vi "OOP_test_main.vi"() -> ()   [LabVIEW 2013]
doc: "Main test automation program using object-oriented programming approach and a producer-consumer architecture."
uses:
  Classes/BaseProducer/IO Task Cluster.ctl
  Classes/BaseProducer/BaseProducer.lvclass
  Classes/BaseProducer/BaseProducer.lvclass/BaseProducer.ctl
panel:
  in  "Stop Button":bool
  in  "Abort":bool
  in  "Front Panel":T1(tab)
  in  "connection information":string="mySQL measurement data"
  in  "Initialize":bool
  in  "test state file path":path=path "C:/Users/Nathan/Documents/LV_testRig-Git/Data/state_sequence_10.txt"
  in  "table":string="10_op_point_test"
  in  "columns":string[](array[string])=["atmosphericP", "opPointDes", "opPointAct", "flameStatus", "dateTimeStamp", "staticP", "temperature", "dynamicP"]
  in  "IO Task Cluster":T2={"Dynamic P Tasks"="DynP_all_S6AI0-4", "AI Tasks"="AiTasks_TC_P_S3", "DIO Tasks"="MFCOutputEnable_S2P0L67", "AO Tasks"="MFCVoltageOut_S2AO0-3"}
  in  "Username":string="Nathan"
  in  "Password":string="admin"
  out "P ATM (psi abs)":dbl=14.424752317565863
  in  "Set P ATM":bool
  in  "Run":bool caption="Run Experiment"
  in  "Measure time (sec)":dbl=1.0
  in  "Back to Default":bool
  out "Remaining":dbl=1181.1679229736328 caption="Time Remaining (sec)"
  in  "End Cooldown":bool
  out "Relight Point":dbl[](array[numeric])=[0.7, 0.0, 2.0, 0.0]
  out "Des. Op. Pt.":dbl[](array[numeric]) caption="Des. Operating Point"
  out "Flame?":bool=TRUE
  out "Temperature Array (C)":dbl[](array[numeric])=[237.25402836473043, 230.0152646954811, 224.8556597910292, 144.771153562919, 153.15861192981532]
  out "Last Line Read":i16=11
  # "Flow Temp"
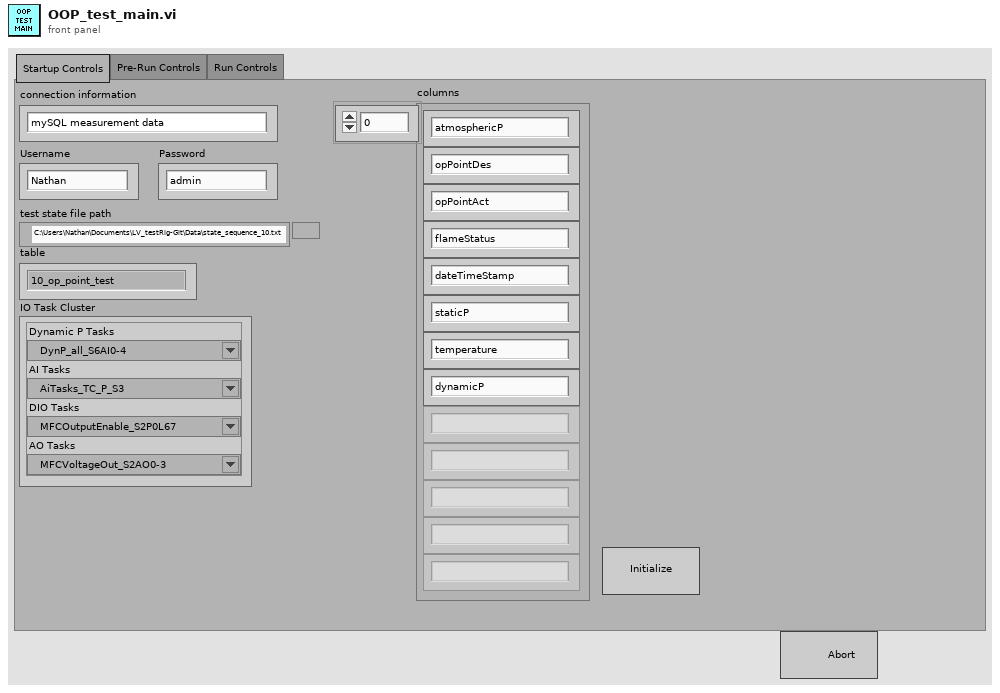
[diagram p1: front panel]
types:
  T1 = enum32{"Startup Controls", "Pre-Run Controls", "Run Controls"}
  T2 = typedef "BaseProducer.lvclass/IO Task Cluster.ctl" = cluster{"Dynamic P Tasks":refnum<k21>, "AI Tasks":refnum<k21>, "DIO Tasks":refnum<k21>, "AO Tasks":refnum<k21>}
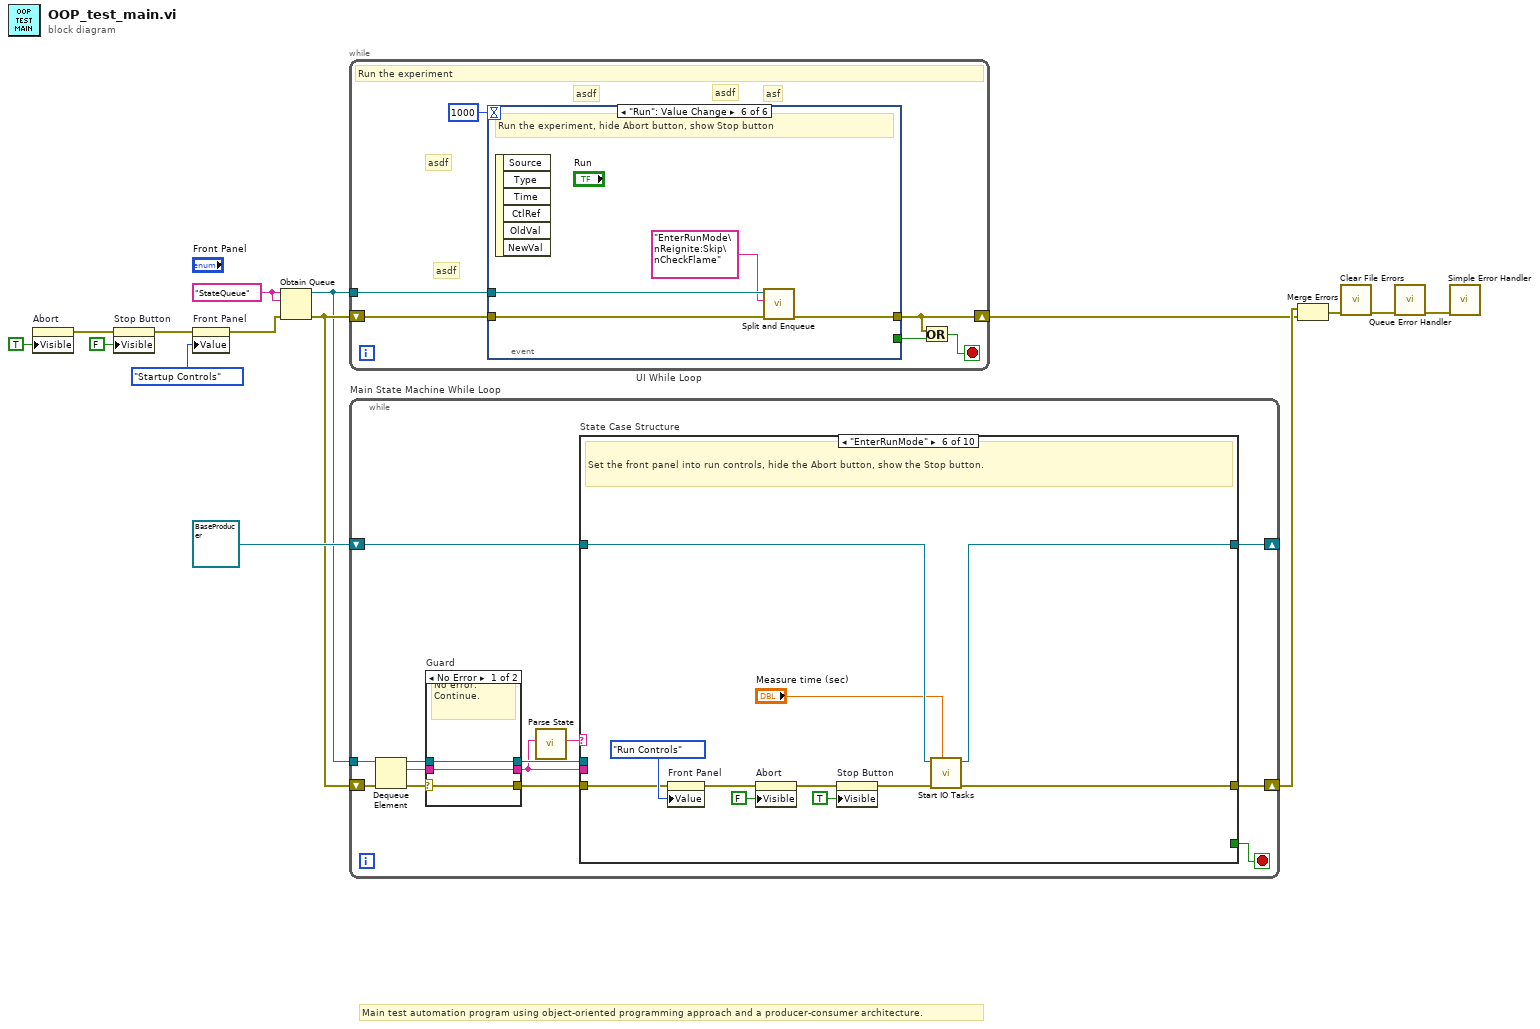
[diagram p0: block diagram]
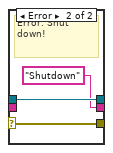
[diagram p2: hidden frame]
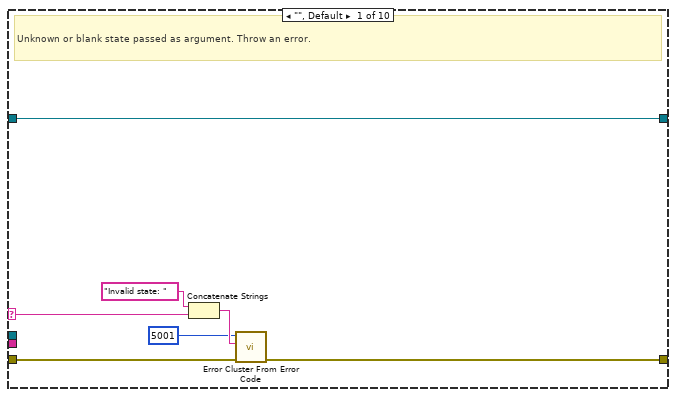
[diagram p3: hidden frame]
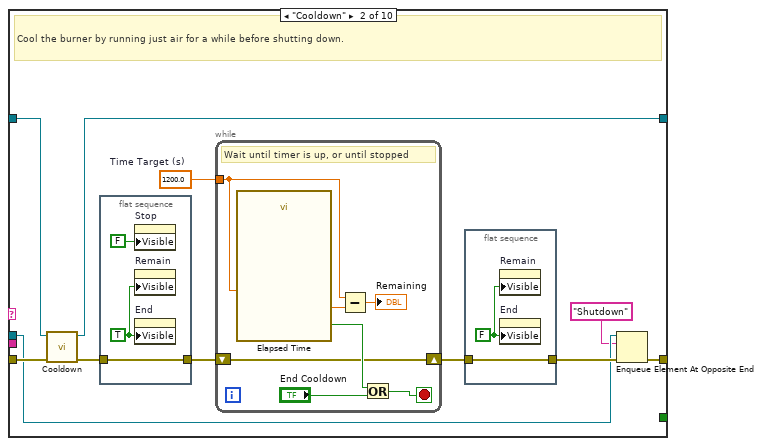
[diagram p4: hidden frame]
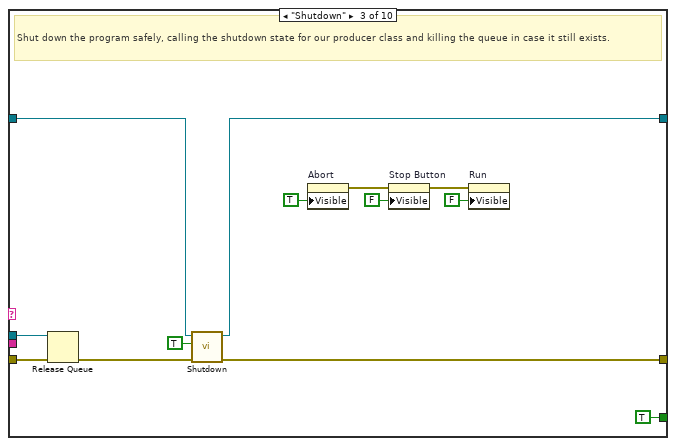
[diagram p5: hidden frame]
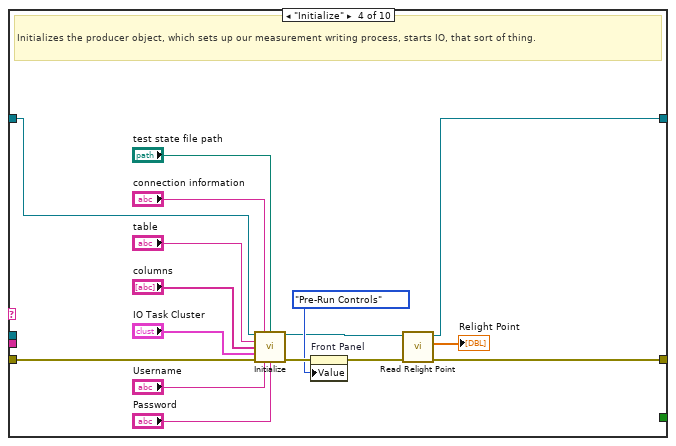
[diagram p6: hidden frame]
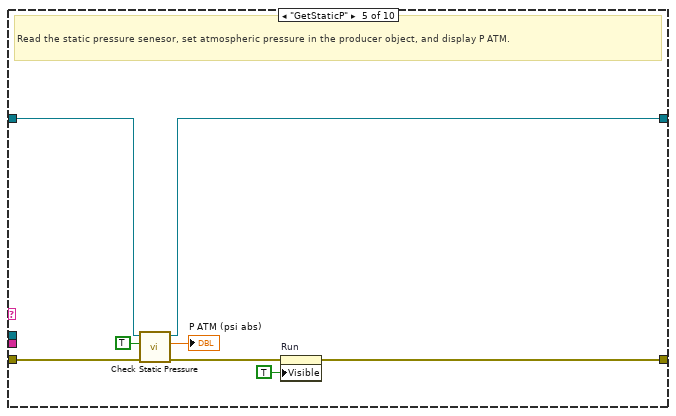
[diagram p7: hidden frame]
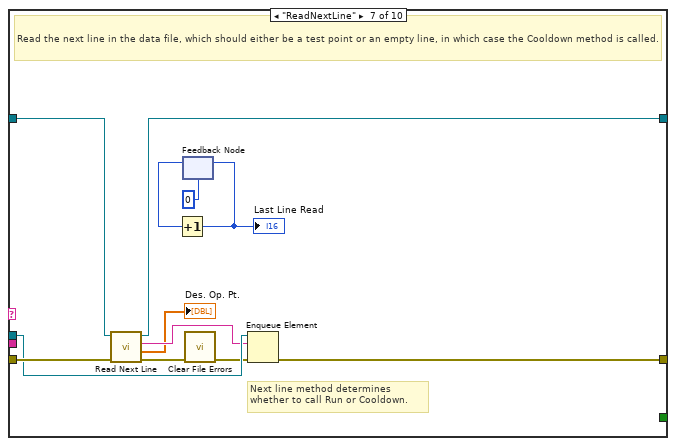
[diagram p8: hidden frame]
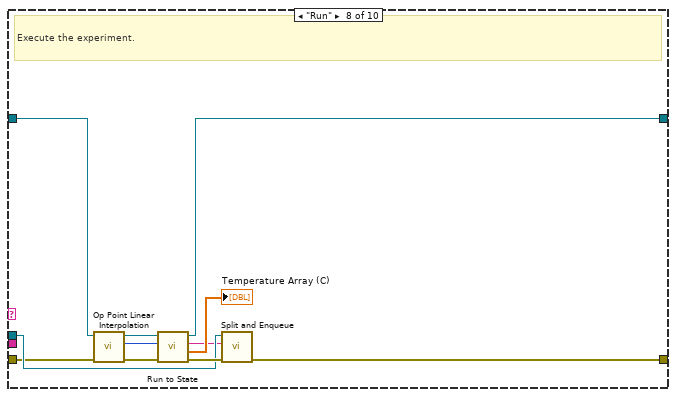
[diagram p9: hidden frame]
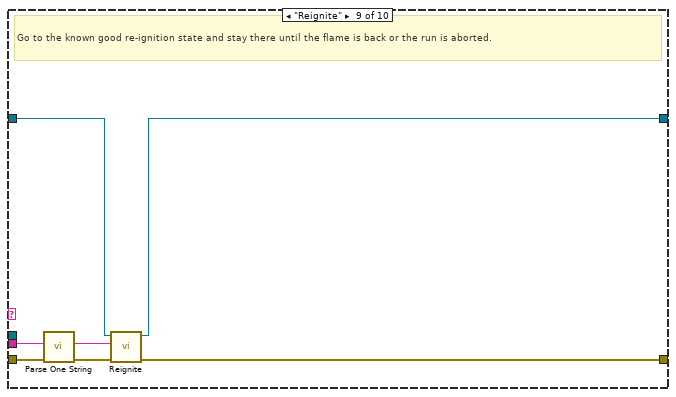
[diagram p10: hidden frame]
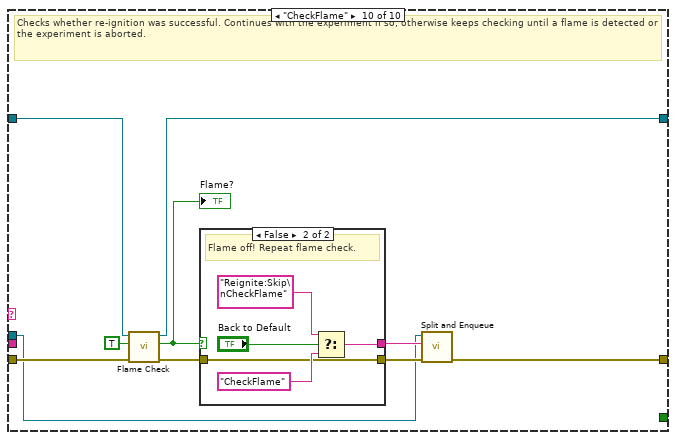
[diagram p11: hidden frame]
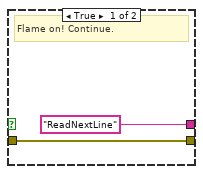
[diagram p12: hidden frame]
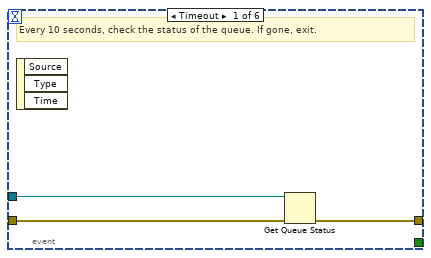
[diagram p13: hidden frame]
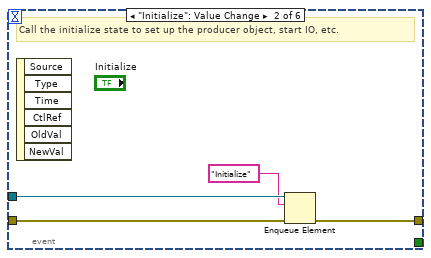
[diagram p14: hidden frame]
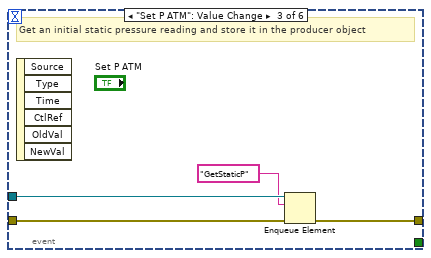
[diagram p15: hidden frame]
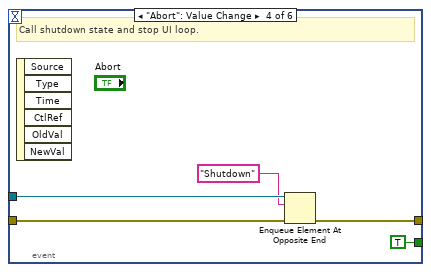
[diagram p16: hidden frame]
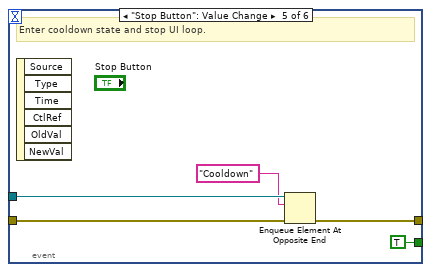
[diagram p17: hidden frame]
diagram:
  w15 = "StateQueue" ("name (unnamed)")
  # "Main test automation program using object-oriented programming approach and a producer-consumer architecture."
  n1 = property on="Abort" class="Bool"("Visible"=TRUE) -> (error out=w9:errorcluster)  [unwired: 2 in, 1 out]
  n2 = property on="Stop Button" class="Bool"(error in=w9, "Visible"=FALSE) -> (error out=w6:errorcluster)  [unwired: 1 in, 1 out]
  n3 = property on="Front Panel" class="TabCtl (strict)"(error in=w6, "Value"=T1."Startup Controls" ("Front Panel")) -> (error out=w11:errorcluster)  [unwired: 1 in, 1 out]
  n4 = Obtain Queue(name (unnamed)=w15, element data type=w15, error in (no error)=w11) -> (queue out=w12:refnum<queue>, error out=w13:errorcluster)  [unwired: 2 in, 1 out]
  n5 = while "UI While Loop" {
    shift-right: [w18] -> w1
    shift-left: w13 -> [w21]
    tunnel: w12 -> [w20]
    stop <- w17 stop-if-true
    # "asdf"
    # "asdf"
    # "asf"
    # "asdf"
    # "asdf"
    # "Run the experiment"
    n6 = event shown="[5] \"Run\": Value Change" {
      selector: _ -> [_ _ _ _ _ _]
      dyn-events: _ -> [_ _ _ _ _ _]
      timeout: 1000 -> [_ _ _ _ _ _]
      tunnel: [_ _ _ TRUE TRUE _] -> w19
      tunnel: w21 -> [w24 w27 w31 w36 w41 w46]
      tunnel: [w22 w28 w32 w37 w40 w45] -> w18
      tunnel: w20 -> [w23 w26 w30 w35 w39 w44]
      event Timeout {
        # "Every 10 seconds, check the status of the queue. If gone, exit."
        n7 = event-data() -> ()  [unwired: 1 in, 3 out]
        n8 = Get Queue Status(queue=w23, error in (no error)=w24) -> (error out=w22:errorcluster)  [unwired: 1 in, 7 out]
      }
      event "Initialize": Value Change {
        # "Call the initialize state to set up the producer object, start IO, etc."
        n9 = event-data() -> ()  [unwired: 1 in, 6 out]
        n10 = Enqueue Element(queue=w26, element="Initialize", error in (no error)=w27) -> (error out=w28:errorcluster)  [unwired: 1 in, 2 out]
      }
      event "Set P ATM": Value Change {
        # "Get an initial static pressure reading and store it in the producer object"
        n11 = event-data() -> ()  [unwired: 1 in, 6 out]
        n12 = Enqueue Element(queue=w30, element="GetStaticP", error in (no error)=w31) -> (error out=w32:errorcluster)  [unwired: 1 in, 2 out]
      }
      event "Abort": Value Change {
        # "Call shutdown state and stop UI loop."
        n13 = event-data() -> ()  [unwired: 1 in, 6 out]
        n14 = Enqueue Element At Opposite End(queue=w35, element="Shutdown", error in (no error)=w36) -> (error out=w37:errorcluster)  [unwired: 1 in, 2 out]
      }
      event "Stop Button": Value Change {
        # "Enter cooldown state and stop UI loop."
        n15 = event-data() -> ()  [unwired: 1 in, 6 out]
        n16 = Enqueue Element At Opposite End(queue=w39, element="Cooldown" ("Input String"), error in (no error)=w41) -> (error out=w40:errorcluster)  [unwired: 1 in, 2 out]
      }
      event "Run": Value Change {
        # "Run the experiment, hide Abort button, show Stop button"
        n17 = event-data() -> ()  [unwired: 1 in, 6 out]
        n18 = call "Split and Enqueue.vi"("error in (no error)"=w46, "Input String"="EnterRunMode\nReignite:Skip\nCheckFlame", "queue in"=w44) -> ("error out"=w45:errorcluster)  [unwired: 7 in, 1 out]
      }
    }
    n19 = Or(x=w18, y=w19) -> (x .or. y?=w17:bool)
  }
  n20 = while "Main State Machine While Loop" {
    shift-right: [w51] -> w2
    shift-left: w13 -> [w59]
    tunnel: w12 -> [w57]
    shift-right: [w48] -> _
    shift-left: refnum<class "BaseProducer.lvclass"> refnum ("BaseProducer.lvclass") -> [w49]
    stop <- w50 stop-if-true
    n21 = Dequeue Element(queue=w57, error in (no error)=w59) -> (queue out=w55:refnum<queue>, element=w56:string, error out=w58:errorcluster)  [unwired: 1 in, 1 out]
    n22 = case "Guard" shown="No Error" w58 {
      selector: w58 -> [w62 w65]
      tunnel: [w62 w65] -> w53
      tunnel: w56 -> [w61 _]
      tunnel: [w61 "Shutdown" ("name (unnamed)")] -> w47
      tunnel: w55 -> [w60 w64]
      tunnel: [w60 w64] -> w54
      frame No Error {
        # "No error. Continue."
      }
      frame Error {
        # "Error. Shut down!"
      }
    }
    n23 = call "Parse State.vi"("String with Args"=w47) -> ("State"=w52:string)  [unwired: 10 in]
    n24 = case "State Case Structure" shown="\"EnterRunMode\"" w52 {
      selector: w52 -> [w68 _ _ _ _ _ _ _ _ _]
      tunnel: w54 -> [_ w76 w105 _ _ _ w153 w162 _ w173]
      tunnel: w53 -> [w69 w82 w108 w121 w132 w142 w155 w160 w172 w178]
      tunnel: [w67 w77 w99 w114 w127 w135 w144 w163 w170 w175] -> w51
      tunnel: [_ _ TRUE _ _ _ _ _ _ _] -> w50
      tunnel: w49 -> [w66 w74 w104 w120 w131 w136 w154 w158 w171 w179]
      tunnel: [w66 w73 w96 w112 w125 w134 w145 w166 w169 w177] -> w48
      tunnel: w47 -> [_ _ _ _ _ _ _ _ w168 _]
      frame "", Default {
        # "Unknown or blank state passed as argument. Throw an error."
        n25 = Concatenate Strings("Invalid state: " ("string"), w68) -> (w71:string)
        n26 = call <vilib>:"Error Cluster From Error Code.vi"("error in (no error)"=w69, "error message (\"\")"=w71, "error code (0)"=5001) -> ("error out"=w67:errorcluster)  [unwired: 6 in]
      }
      frame "Cooldown" {
        w83 = 1200.0  # Time Target (s)
        # "Cool the burner by running just air for a while before shutting down."
        n27 = call "Cooldown.vi"("error in (no error)"=w82, "BaseProducer in"=w74) -> ("error out"=w81:errorcluster, "BaseProducer out"=w73:refnum<class "BaseProducer.lvclass">)  [unwired: 7 in, 1 out]
        n28 = flat-sequence {
          tunnel: w81 -> [w88]
          tunnel: [w88] -> w80
          frame #0 {
            w87 = TRUE ("Visible")
            n29 = property on="Stop" class="Bool"("Visible"=FALSE) -> ()  [unwired: 2 in, 2 out]
            n30 = property on="Remain" class="DigNum (strict)"("Visible"=w87) -> ()  [unwired: 2 in, 2 out]
            n31 = property on="End" class="Bool"("Visible"=w87) -> ()  [unwired: 2 in, 2 out]
          }
        }
        n32 = while {
          tunnel: w83 -> [w94]
          shift-right: [w90] -> w79
          shift-left: w80 -> [w90]
          stop <- w89 stop-if-true
          # "Wait until timer is up, or until stopped"
          n33 = call "Elapsed Time"("Time Target (s)"=w94) -> ("Elapsed Time (s)"=w95:dbl, "Time has Elapsed"=w91:bool)  [unwired: 11 in, 6 out]
          n34 = Subtract(x=w94, y=w95) -> (x-y=→"Remaining":dbl)
          n35 = Or(x=w91, y="End Cooldown") -> (x .or. y?=w89:bool)
        }
        n36 = flat-sequence {
          tunnel: w79 -> [w85]
          tunnel: [w85] -> w78
          frame #0 {
            w84 = FALSE ("Visible")
            n37 = property on="Remain" class="DigNum (strict)"("Visible"=w84) -> ()  [unwired: 2 in, 2 out]
            n38 = property on="End" class="Bool"("Visible"=w84) -> ()  [unwired: 2 in, 2 out]
          }
        }
        n39 = Enqueue Element At Opposite End(queue=w76, element="Shutdown", error in (no error)=w78) -> (error out=w77:errorcluster)  [unwired: 1 in, 2 out]
      }
      frame "Shutdown" {
        # "Shut down the program safely, calling the shutdown state for our producer class and killing the queue in case it still exists."
        n40 = Release Queue(queue=w105, error in (no error)=w108) -> (error out=w106:errorcluster)  [unwired: 1 in, 2 out]
        n41 = call "Shutdown.vi"("error in (no error)"=w106, "Kill Now? (T)"=TRUE, "BaseProducer in"=w104) -> ("error out"=w99:errorcluster, "BaseProducer out"=w96:refnum<class "BaseProducer.lvclass">)  [unwired: 7 in]
        n42 = property on="Abort" class="Bool"("Visible"=TRUE) -> (error out=w100:errorcluster)  [unwired: 2 in, 1 out]
        n43 = property on="Stop Button" class="Bool"(error in=w100, "Visible"=FALSE) -> (error out=w98:errorcluster)  [unwired: 1 in, 1 out]
        n44 = property on="Run" class="Bool"(error in=w98, "Visible"=FALSE) -> ()  [unwired: 1 in, 2 out]
      }
      frame "Initialize" {
        # "Initializes the producer object, which sets up our measurement writing process, starts IO, that sort of thing."
        n45 = call "Initialize.vi"("BaseProducer in"=w120, "connection information"="connection information", "test state file path"="test state file path", "table"="table", "columns"="columns", "IO Task Cluster"="IO Task Cluster", "error in (no error)"=w121, "Username"="Username", "Password"="Password") -> ("BaseProducer out"=w115:refnum<class "BaseProducer.lvclass">, "error out"=w124:errorcluster)  [unwired: 5 in]
        n46 = property on="Front Panel" class="TabCtl (strict)"(error in=w124, "Value"=T1."Pre-Run Controls" ("Front Panel")) -> (error out=w116:errorcluster)  [unwired: 1 in, 1 out]
        n47 = call "Read Relight Point.vi"("error in (no error)"=w116, "BaseProducer in"=w115) -> ("error out"=w114:errorcluster, "Relight Point"=→"Relight Point":dbl[], "BaseProducer out"=w112:refnum<class "BaseProducer.lvclass">)  [unwired: 7 in]
      }
      frame "GetStaticP" {
        # "Read the static pressure senesor, set atmospheric pressure in the producer object, and display P ATM."
        n48 = call "Check Static Pressure.vi"("error in (no error)"=w132, "Set P ATM? (F)"=TRUE, "BaseProducer in"=w131) -> ("error out"=w128:errorcluster, "Pressure (psi atm)"=→"P ATM (psi abs)":dbl, "BaseProducer out"=w125:refnum<class "BaseProducer.lvclass">)  [unwired: 6 in]
        n49 = property on="Run" class="Bool"(error in=w128, "Visible"=TRUE) -> (error out=w127:errorcluster)  [unwired: 1 in, 1 out]
      }
      frame "EnterRunMode" {
        # "Set the front panel into run controls, hide the Abort button, show the Stop button."
        n50 = property on="Front Panel" class="TabCtl (strict)"(error in=w142, "Value"=T1."Run Controls" ("Front Panel")) -> (error out=w141:errorcluster)  [unwired: 1 in, 1 out]
        n51 = property on="Abort" class="Bool"(error in=w141, "Visible"=FALSE) -> (error out=w139:errorcluster)  [unwired: 1 in, 1 out]
        n52 = property on="Stop Button" class="Bool"(error in=w139, "Visible"=TRUE) -> (error out=w137:errorcluster)  [unwired: 1 in, 1 out]
        n53 = call "Start IO Tasks.vi"("Measure time (sec)"="Measure time (sec)", "error in (no error)"=w137, "BaseProducer in"=w136) -> ("error out"=w135:errorcluster, "BaseProducer out"=w134:refnum<class "BaseProducer.lvclass">)  [unwired: 7 in]
      }
      frame "ReadNextLine" {
        # "Next line method determines\nwhether to call Run or Cooldown."
        # "Read the next line in the data file, which should either be a test point or an empty line, in which case the Cooldown method is called."
        n54 = call "Read Next Line.vi"("error in (no error)"=w155, "BaseProducer in"=w154) -> ("error out"=w149:errorcluster, "Operating Point"=→"Des. Op. Pt.":dbl[], "Next State"=w147:string, "BaseProducer out"=w145:refnum<class "BaseProducer.lvclass">)  [unwired: 6 in]
        n55 = feedback #1(i16 0) -> (w151:i16)
        n56 = Increment(x=w151) -> (x+1=w150:i16)
        "Last Line Read" <- w150
        n57 = feedback-in #1(w150) -> ()
        n58 = call "Clear File Errors.vi"("Error In"=w149) -> ("Error Out"=w148:errorcluster)  [unwired: 10 in]
        n59 = Enqueue Element(queue=w153, element=w147, error in (no error)=w148) -> (error out=w144:errorcluster)  [unwired: 1 in, 2 out]
      }
      frame "Run" {
        # "Execute the experiment."
        n60 = call "Op Point Linear Interpolation.vi"("error in (no error)"=w160, "BaseProducer in"=w158) -> ("error out"=w159:errorcluster, "Num moves"=w156:i32, "BaseProducer out"=w157:refnum<class "BaseProducer.lvclass">)  [unwired: 7 in]
        n61 = call "Run to State.vi"("error in (no error)"=w159, "Num moves"=w156, "BaseProducer in"=w157) -> ("error out"=w164:errorcluster, "Temperature Array (C)"=→"Temperature Array (C)":dbl[], "Next State"=w161:string, "BaseProducer out"=w166:refnum<class "BaseProducer.lvclass">)  [unwired: 5 in]
        n62 = call "Split and Enqueue.vi"("error in (no error)"=w164, "Input String"=w161, "queue in"=w162) -> ("error out"=w163:errorcluster)  [unwired: 7 in, 1 out]
      }
      frame "Reignite" {
        # "Go to the known good re-ignition state and stay there until the flame is back or the run is aborted."
        n63 = call "Parse One String.vi"("State String"=w168) -> ("Argument"=w167:string)  [unwired: 10 in]
        n64 = call "Reignite.vi"("error in (no error)"=w172, "Relight State"=w167, "BaseProducer in"=w171) -> ("error out"=w170:errorcluster, "BaseProducer out"=w169:refnum<class "BaseProducer.lvclass">)  [unwired: 7 in]
      }
      frame "CheckFlame" {
        # "Checks whether re-ignition was successful. Continues with the experiment if so, otherwise keeps checking until a flame is detected or the experiment is aborted."
        n65 = call "Flame Check.vi"("error in (no error)"=w178, "Resample? (F)"=TRUE, "BaseProducer in"=w179) -> ("error out"=w182:errorcluster, "Flame?"=w181:bool, "BaseProducer out"=w177:refnum<class "BaseProducer.lvclass">)  [unwired: 6 in]
        "Flame?" <- w181
        n66 = case shown="False" w181 {
          tunnel: w182 -> [w184 w186]
          tunnel: [w184 w186] -> w176
          tunnel: ["ReadNextLine" ("element") w185] -> w174
          frame True {
            # "Flame on! Continue."
          }
          frame False {
            # "Flame off! Repeat flame check."
            n67 = Select(t="Reignite:Skip\nCheckFlame" ("element"), s="Back to Default", f="CheckFlame" ("element")) -> (s? t:f=w185:string)
          }
        }
        n68 = call "Split and Enqueue.vi"("error in (no error)"=w176, "Input String"=w174, "queue in"=w173) -> ("error out"=w175:errorcluster)  [unwired: 7 in, 1 out]
      }
    }
  }
  n69 = Merge Errors(w2, w1) -> (w4:errorcluster)
  n70 = call "Clear File Errors.vi"("Error In"=w4) -> ("Error Out"=w5:errorcluster)  [unwired: 10 in]
  n71 = call "Queue Error Handler.vi"("Error In"=w5) -> ("Error Out"=w3:errorcluster)  [unwired: 10 in]
  n72 = call <vilib>:"Simple Error Handler.vi"("error in (no error)"=w3) -> ()  [unwired: 4 in, 5 out]
